vi "Sort Schedules.vi"(11 "Schedules":T1[](array[typedef])) -> (3 "sorted Schedules":T1[](array[typedef]))   [LabVIEW 2017, in "DSF Core.lvlib" / "Scheduler.lvclass"]
uses:
  Scheduler.lvclass
  Transfer Group Scheduler Data.ctl
  Timing/Timing.lvclass
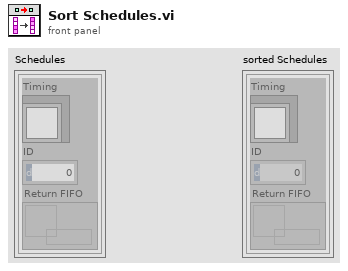
[diagram p1: front panel]
types:
  T1 = typedef "DSF Core.lvlib/Scheduler.lvclass/Transfer Group Scheduler Data.ctl" = cluster{"Timing":refnum<class "Timing.lvclass">, "ID":i32, "Return FIFO":refnum<k33>}
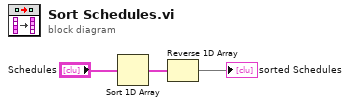
[diagram p0: block diagram]
diagram:
  n1 = Sort 1D Array(array="Schedules") -> (sorted array=w2:T1[])
  n2 = Reverse 1D Array(array=w2) -> (reversed array=→"sorted Schedules":T1[])
